vi "Chroma2.vi"() -> ()   [LabVIEW 2015]
uses:
  <vilib>/Utility/file.llb/Write To Spreadsheet File (string).vi
panel:
  in  "Press to Stop":bool
  out "error out":errorcluster
  in  "Name of File":string
  out "Current Data Point":i32
  in  "Type (P_REAL)":i32(ring) items=["P_ENERGY"=4, "P_FACTOR"=3, "P_REACTIVE"=2, "P_APPARENT"=1, "P_REAL"=0]
  in  "Type (I_RMS)":i32(ring) items=["I_THD"=5, "I_CRESTFACTOR"=4, "I_INRUSH"=3, "I_PEAK-"=2, "I_PEAK+"=1, "I_RMS"=0]
  in  "Type (V_RMS)":i32(ring) items=["V_THD"=3, "V_PEAK-"=2, "V_PEAK+"=1, "V_RMS"=0]
  in  "Port Name":refnum<visa-resource-name> caption="resource name"
  # "CHROMA"
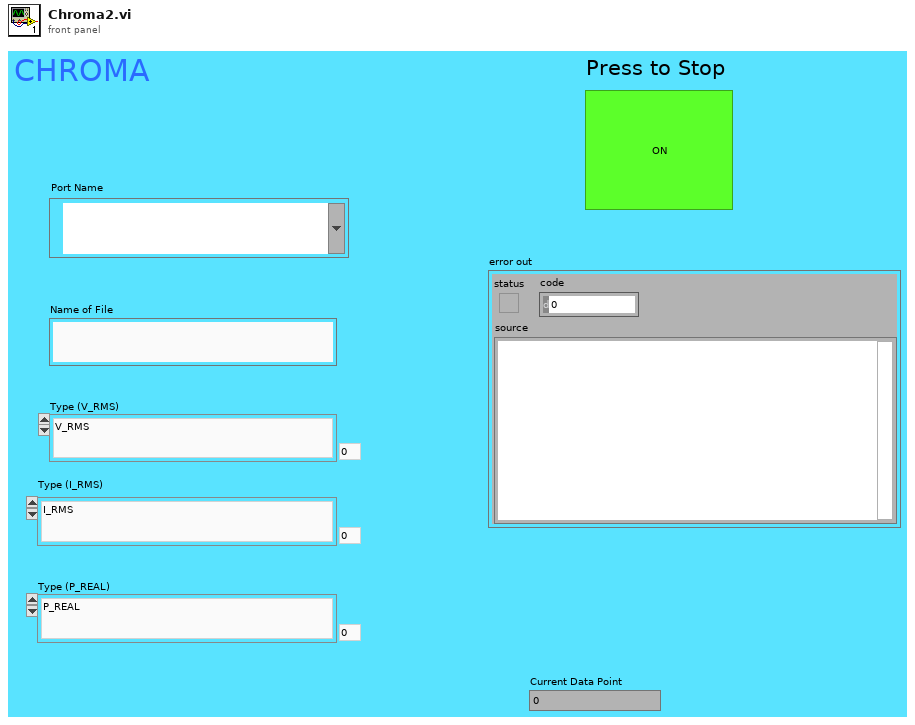
[diagram p1: front panel]
types:
  T1 = enum16{"open", "replace", "create", "open or create", "replace or create", "replace or create with confirmation"}
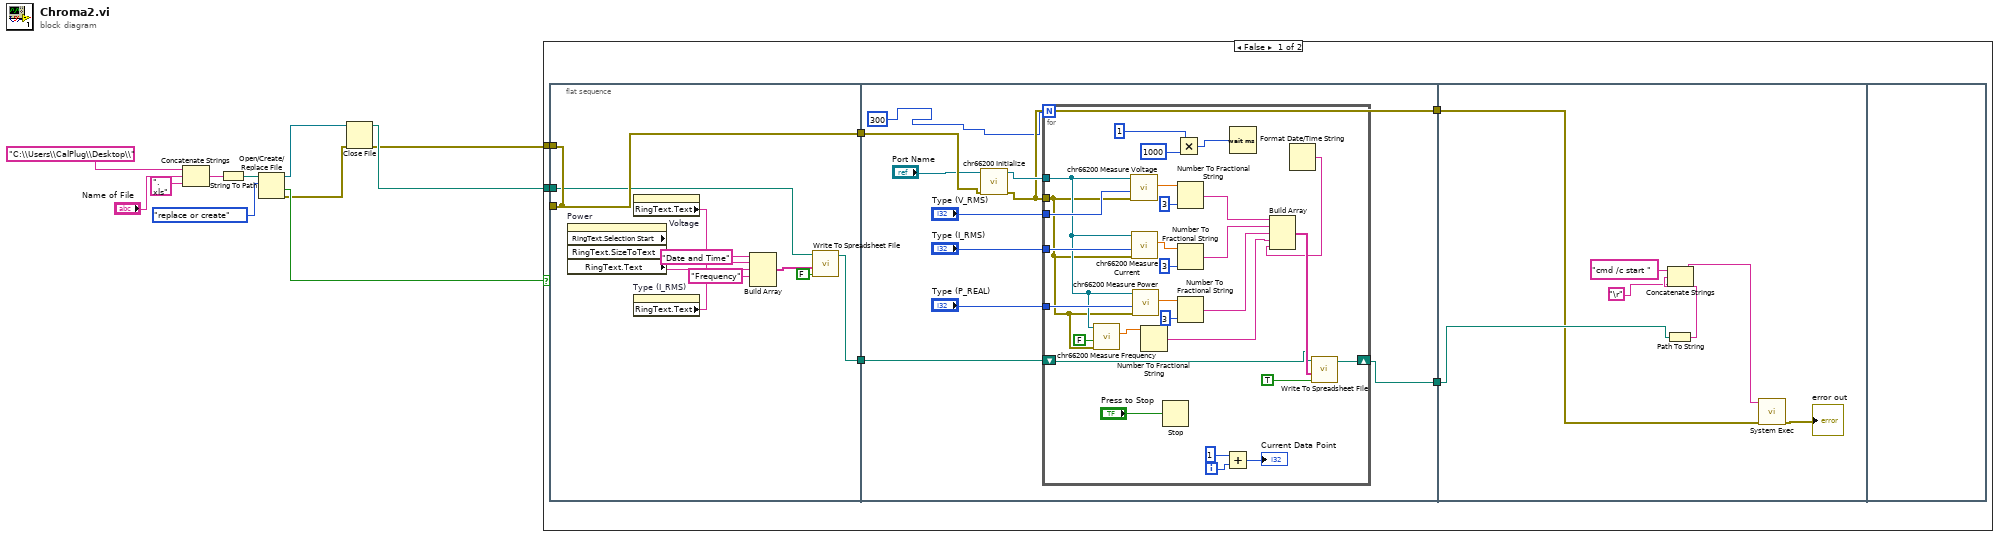
[diagram p0: block diagram]
diagram:
  n1 = Concatenate Strings("C:\\Users\\CalPlug\\Desktop\\" ("string"), "Name of File", ".xls" ("string")) -> (w11:string)
  n2 = String To Path(string=w11) -> (path=w10:path)
  n3 = Open/Create/Replace File(file path (use dialog)=w10, operation (0:open)=T1."replace or create") -> (refnum out=w4:refnum<file>, cancelled=w5:bool, error out=w2:errorcluster)  [unwired: 4 in]
  n4 = Close File(refnum=w4, error in=w2) -> (path=w3:path, error out=w1:errorcluster)
  n5 = case shown="False" w5 {
    tunnel: w3 -> [w15 _]
    tunnel: w1 -> [w12 _]
    frame False {
      n6 = flat-sequence {
        tunnel: [w27] -> w17
        tunnel: [w20] -> w16
        tunnel: [w20] -> _
        tunnel: w15 -> [w19]
        tunnel: w12 -> [w20]
        tunnel: w17 -> [w31]
        tunnel: w16 -> [w33]
        tunnel: [w32] -> w14
        tunnel: [w30] -> w13
        tunnel: w14 -> [w72]
        tunnel: w13 -> [w67]
        frame #0 {
          n7 = property on="Power" class="Ring (strict)" props=["RingText", "Selection Start", "RingText", "SizeToText", "RingText", "Text"]() -> ("RingText.Text"=w24:string)  [unwired: 2 in, 4 out]
          n8 = property on="Voltage" class="Ring (strict)"() -> ("RingText.Text"=w25:string)  [unwired: 2 in, 2 out]
          n9 = property on="Type (I_RMS)" class="Ring (strict)"() -> ("RingText.Text"=w23:string)  [unwired: 2 in, 2 out]
          n10 = Build Array(w25, w23, w24, "Frequency" ("element"), "Date and Time" ("element")) -> (w22:string[])
          n11 = call-poly <vilib>:"Write To Spreadsheet File.vi"("append to file? (new file:F)"=FALSE, "1D data"=w22, "file path (dialog if empty)"=w19) -> ("new file path (Not A Path if cancelled)"=w27:path)  [unwired: 5 in]
        }
        frame #1 {
          n12 = call <instrlib>:"chr66200 Initialize.vi"("error in (no error)"=w33, "resource name"="Port Name") -> ("error out"=w30:errorcluster, "instrument handle out"=w34:refnum<k15>)  [unwired: 8 in]
          n13 = for {
            N: u32 300 ("seconds to wait") -> [_]
            tunnel: w34 -> [w47]
            tunnel: w30 -> [w42]
            tunnel: "Type (I_RMS)" -> [w66]
            tunnel: "Type (V_RMS)" -> [w65]
            tunnel: "Type (P_REAL)" -> [w64]
            shift-right: [w63] -> w32
            shift-left: w31 -> [w41]
            i -> [w54]
            n14 = call <instrlib>:"chr66200 Measure Frequency.vi"("error in (no error)"=w42, 9:FALSE ("Measure Fetch (Fetch)"), "instrument handle"=w47) -> ("Read Value"=w45:dbl)  [unwired: 6 in, 2 out]
            n15 = call <instrlib>:"chr66200 Measure Voltage.vi"("error in (no error)"=w42, "Type (V_RMS)"=w65, "instrument handle"=w47) -> ("Read Value"=w61:dbl)  [unwired: 6 in, 2 out]
            n16 = call <instrlib>:"chr66200 Measure Current.vi"("error in (no error)"=w42, "Type (I_RMS)"=w66, "instrument handle"=w47) -> ("Read Value"=w60:dbl)  [unwired: 6 in, 2 out]
            n17 = call <instrlib>:"chr66200 Measure Power.vi"("error in (no error)"=w42, "Type (P_REAL)"=w64, "instrument handle"=w47) -> ("Read Value"=w59:dbl)  [unwired: 6 in, 2 out]
            n18 = Number To Fractional String(number=w45) -> (F-format string=w43:string)  [unwired: 3 in]
            n19 = Stop(stop? (T)="Press to Stop") -> ()
            n20 = Multiply(x=u32 1 ("Interval of Data Collection (sec)"), y=u32 1000) -> (x*y=w50:u32)
            n21 = Number To Fractional String(number=w61, precision (6)=i16 3) -> (F-format string=w49:string)  [unwired: 2 in]
            n22 = Number To Fractional String(number=w60, precision (6)=i16 3) -> (F-format string=w48:string)  [unwired: 2 in]
            n23 = Number To Fractional String(number=w59, precision (6)=i16 3) -> (F-format string=w44:string)  [unwired: 2 in]
            n24 = Add(x=1, y=w54) -> (x+y=→"Current Data Point":i32)
            n25 = Wait (ms)(milliseconds to wait=w50) -> ()  [unwired: 1 out]
            n26 = Format Date/Time String() -> (date/time string=w38:string)  [unwired: 3 in]
            n27 = Build Array(w49, w48, w44, w43, w38) -> (w55:string[])
            n28 = call-poly <vilib>:"Write To Spreadsheet File.vi"("append to file? (new file:F)"=TRUE, "1D data"=w55, "file path (dialog if empty)"=w41) -> ("new file path (Not A Path if cancelled)"=w63:path)  [unwired: 5 in]
          }
        }
        frame #2 {
          n29 = Path To String(path=w72) -> (string=w71:string)
          n30 = Concatenate Strings("cmd /c start " ("string"), w71, "\r") -> (w69:string)
          n31 = call <vilib>:"System Exec.vi"("error in (no error)"=w67, "command line"=w69) -> ("error out"=→"error out":errorcluster)  [unwired: 6 in, 3 out]
        }
        frame #3 {
        }
      }
    }
    frame True {
    }
  }
